vi "Configure.vi"(0 "ADChannel":i32(ring) items=["Disabled", "CH1 Enabled", "CH2 Enabled", "Both Enabled"], 1 "ADSampleRate":i32(ring)=100000 items=["450Ksps"=450000, "250Ksps"=250000, "100Ksps"=100000, "50Ksps"=50000, "25Ksps"=25000, "10Ksps"=10000, "5Ksps"=5000, "2Ksps"=2000, "1Ksps"=1000], 2 "GainIndex":i32(ring) items=["Gain = 1", "Gain = 2", "Gain = 5", "Gain = 10"], 4 "DeviceHandle":i32) -> (5 "Error":bool)   [LabVIEW 2012]
uses:
  MPS-060602.dll
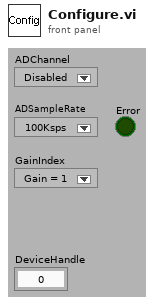
[diagram p1: front panel]
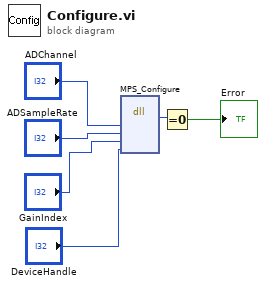
[diagram p0: block diagram]
diagram:
  n1 = dll-call lib="PTH1Yabs CDocuments and Settings\nAdministrator桌面性能\tdriver VIMPS-060602.dll" fn="MPS_Configure"("ADChannel"="ADChannel", "ADSampleRate"="ADSampleRate", "GainIndex"="GainIndex", "DeviceHandle"="DeviceHandle") -> (w2:i32)  [unwired: 7 in, 2 out]
  n2 = Equal To 0?(x=w2) -> (x = 0?=→"Error":bool)
